vi "Lift_State.vi"(9 "Drive Control":T1 {"Power (100)" min=-100 max=100}, 11 "Dump Open":u8) -> ()   [LabVIEW 2012, in "Serenity_mk2.lvrbt"]
uses:
  Serenity_mk2.lvrbt
  auto_drive_TYP.ctl
  <vilib>/NXT/Hardware/Plugins/Tetrix DC Motor/TetrixDCMotorAddress.ctl
  <vilib>/NXT/Hardware/Plugins/Tetrix 180 deg Servo/Tetrix180ServoAddress.ctl
  <vilib>/NXT/NXTIO Xnodes/NXTIONodeSubVIs/TETRIX IO Move DC Motors.vi
  <vilib>/NXT/NXTIO Xnodes/NXTIONodeSubVIs/TETRIX IO Motor Status.vi
  <vilib>/NXT/Dual Mode Library/Sound/Tone.vi
  <vilib>/NXT/NXTIO Xnodes/NXTIONodeSubVIs/TETRIX IO Move Servos.vi
  <vilib>/NXT/NXTIO Xnodes/AddressXNode/NXTIOAddress.xnode
  <vilib>/NXT/Subs/LVHSConnector.ctl
  <vilib>/NXT/NXTIO Xnodes/NXTIOXNode/NXTIO.xnode
  <vilib>/NXT/LegoClasses/BrickReference/BrickReference.lvclass
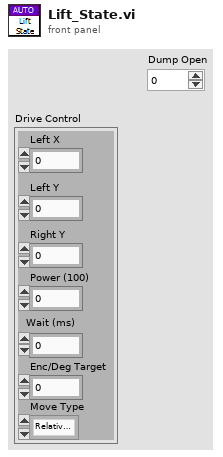
[diagram p1: front panel]
types:
  T1 = typedef "auto_drive_TYP.ctl" = cluster{"Left X":i8, "Left Y":i8, "Right Y":i8, "Power (100)":i8, "Wait (ms)":u32, "Enc/Deg Target":i32, "Move Type":enum16{"Relative Degrees", "Wait", "Encoder"}}
  T2 = typedef "TetrixDCMotorAddress.ctl" = i32
  T3 = typedef "LVHSConnector.ctl" = refnum<class "BrickReference.lvclass">
  T4 = typedef "Tetrix180ServoAddress.ctl" = i32
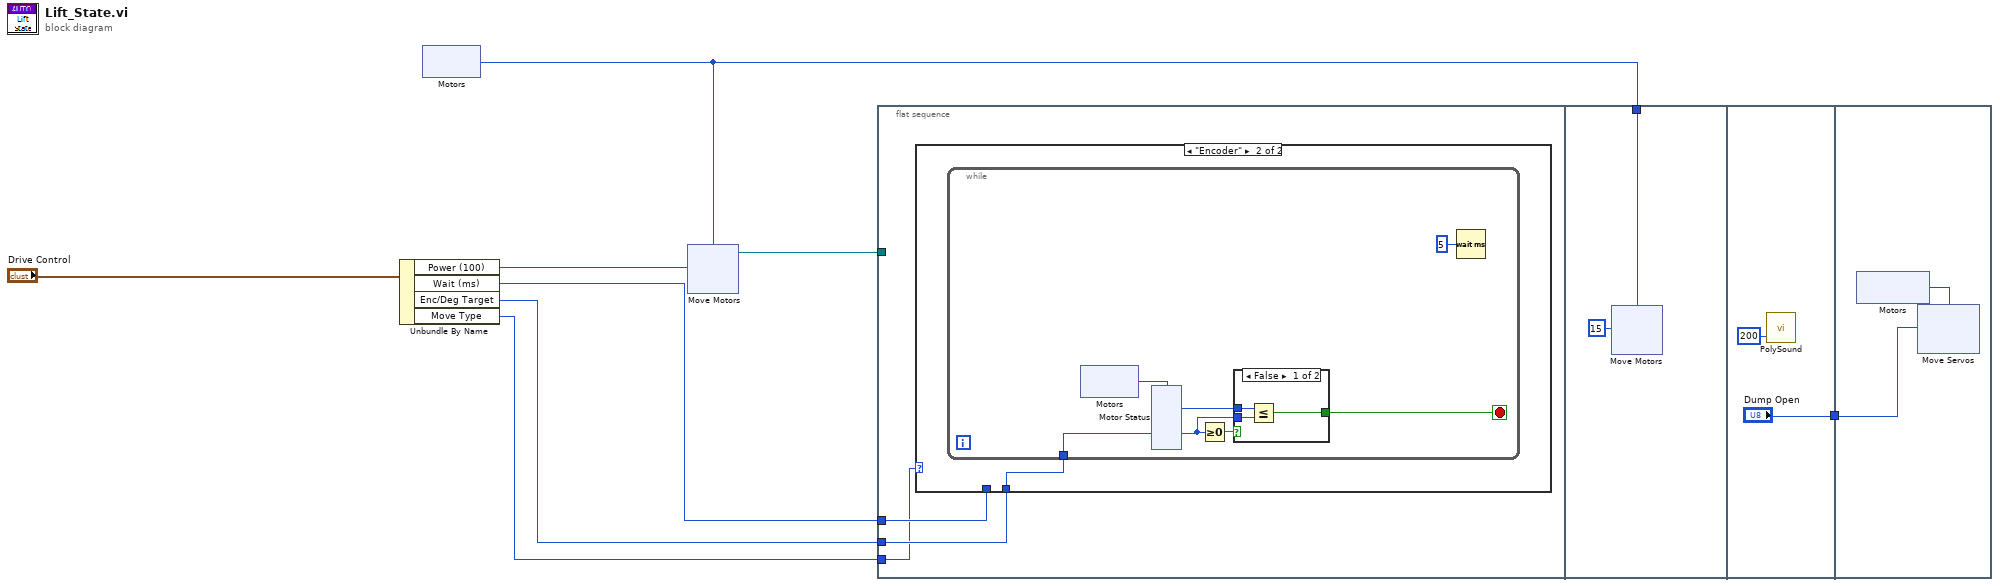
[diagram p0: block diagram]
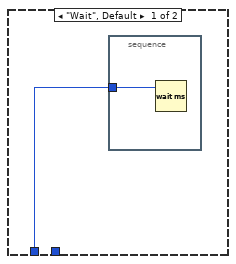
[diagram p2: hidden frame]
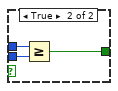
[diagram p3: hidden frame]
diagram:
  n1 = Unbundle By Name("Drive Control") -> ("Power (100)"=w6:i8, "Wait (ms)"=w4:u32, "Enc/Deg Target"=w5:i32, "Move Type"=w8:enum16{"Relative Degrees", "Wait", "Encoder"})
  n2 = xnode "Motors"() -> ("Motor"=w1:T2)
  n3 = xnode "Move Motors"("Power/Speed 1"=w6, "Motors"=w1) -> ("NXT/EV3"=w7:T3)  [unwired: 1 in]
  n4 = flat-sequence {
    tunnel: w4 -> [w11]
    tunnel: w5 -> [w10]
    tunnel: w8 -> [w9]
    tunnel: w7 -> [_]
    tunnel: w1 -> [w36]
    tunnel: ["Dump Open"] -> w2
    tunnel: w2 -> [w47]
    frame #0 {
      n5 = case shown="\"Encoder\"" w9 {
        tunnel: w11 -> [w12 _]
        tunnel: w10 -> [_ w14]
        frame "Wait", Default {
          n6 = stacked-sequence {
            tunnel: w12 -> [w13]
            frame #0 {
              n7 = Wait (ms)(milliseconds to wait=w13) -> ()  [unwired: 1 out]
            }
          }
        }
        frame "Encoder" {
          n8 = while {
            tunnel: w14 -> [w17]
            stop <- w18 stop-if-true
            n9 = xnode "Motors"() -> ("Motor"=w20:T2)
            n10 = xnode "Motor Status"("Motors"=w20) -> ("Position 1"=w16:i32)  [unwired: 1 in, 2 out]
            n11 = Greater Or Equal To 0?(x=w17) -> (x >= 0?=w19:bool)
            n12 = case shown="False" w19 {
              tunnel: w16 -> [w23 w26]
              tunnel: [w21 w25] -> w18
              tunnel: w17 -> [w22 w24]
              frame False {
                n13 = Less Or Equal?(x=w23, y=w22) -> (x <= y?=w21:bool)
              }
              frame True {
                n14 = Greater Or Equal?(x=w26, y=w24) -> (x >= y?=w25:bool)
              }
            }
            n15 = Wait (ms)(milliseconds to wait=u32 5) -> ()  [unwired: 1 out]
          }
        }
      }
    }
    frame #1 {
      n16 = xnode "Move Motors"("Power/Speed 1"=i8 15, "Motors"=w36) -> ()  [unwired: 1 in, 1 out]
    }
    frame #2 {
      n17 = call-poly <vilib>:"PolySound.vi"("Duration (500 ms)"=u16 200) -> ()  [unwired: 3 in, 1 out]
    }
    frame #3 {
      n18 = xnode "Motors"() -> ("Motor"=w48:T4)
      n19 = xnode "Move Servos"("Position 1"=w47, "Motors"=w48) -> ()  [unwired: 1 in, 1 out]
    }
  }
